vi "set_V_channel.vi"(8 "error in (no error)":errorcluster, 11 "Motech-pps-1200 in":refnum<class "Motech-pps-1200.lvclass">) -> (0 "error out":errorcluster, 3 "Motech-pps-1200 out":refnum<class "Motech-pps-1200.lvclass">)   [LabVIEW 2017, in "Motech-pps-1200.lvclass"]
uses:
  Motech-pps-1200.lvclass
  DC_power_supply.lvclass
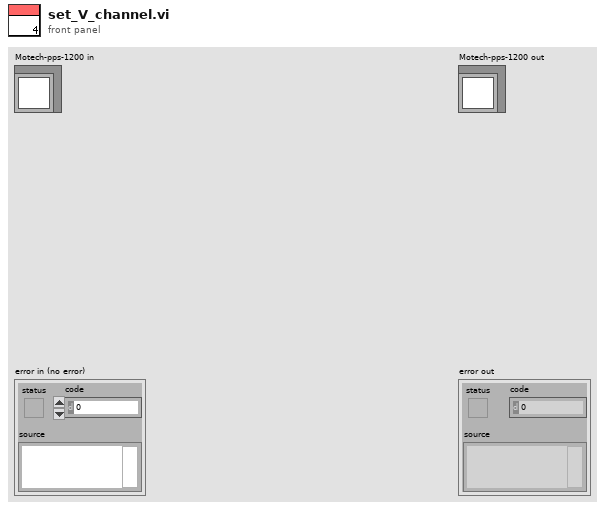
[diagram p1: front panel]
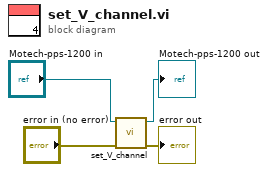
[diagram p0: block diagram]
diagram:
  n1 = call-parent "set_V_channel.vi"("error in (no error)"="error in (no error)", "DC_power_supply in"="Motech-pps-1200 in") -> ("error out"=→"error out":errorcluster, "DC_power_supply out"=→"Motech-pps-1200 out":refnum<class "Motech-pps-1200.lvclass">)  [unwired: 8 in]
